vi "MakePlotDG535.vi"(5 "Polarity array":refnum<vi>[](array[refnum]), 6 "Amplitude array":refnum<vi>[](array[refnum]), 7 "Channel array":refnum<vi>[](array[refnum])) -> (0 "min value":dbl, 1 "Numeric 3":dbl, 2 "samples":i32, 3 "Numeric":T1 min=-999.0 max=999.0 format="%+.12f", 4 "Array":cluster{"Pulse Pattern":dbl[]}[](array[cluster]))   [LabVIEW 2013]
uses:
  GUI_DG645/DelayControl2.ctl
  <vilib>/Analysis/NI_AALBase.lvlib
panel:
  out "Pulse Pattern":dbl[](graph)
  out "Array 2":cluster{"Waveform Graph":dbl[]}[](array[cluster])
  out "Array 4":T1[](array[typedef]) min=-999.0 max=999.0 format="%+.12f"
  out "Array 3":dbl[](array[numeric])
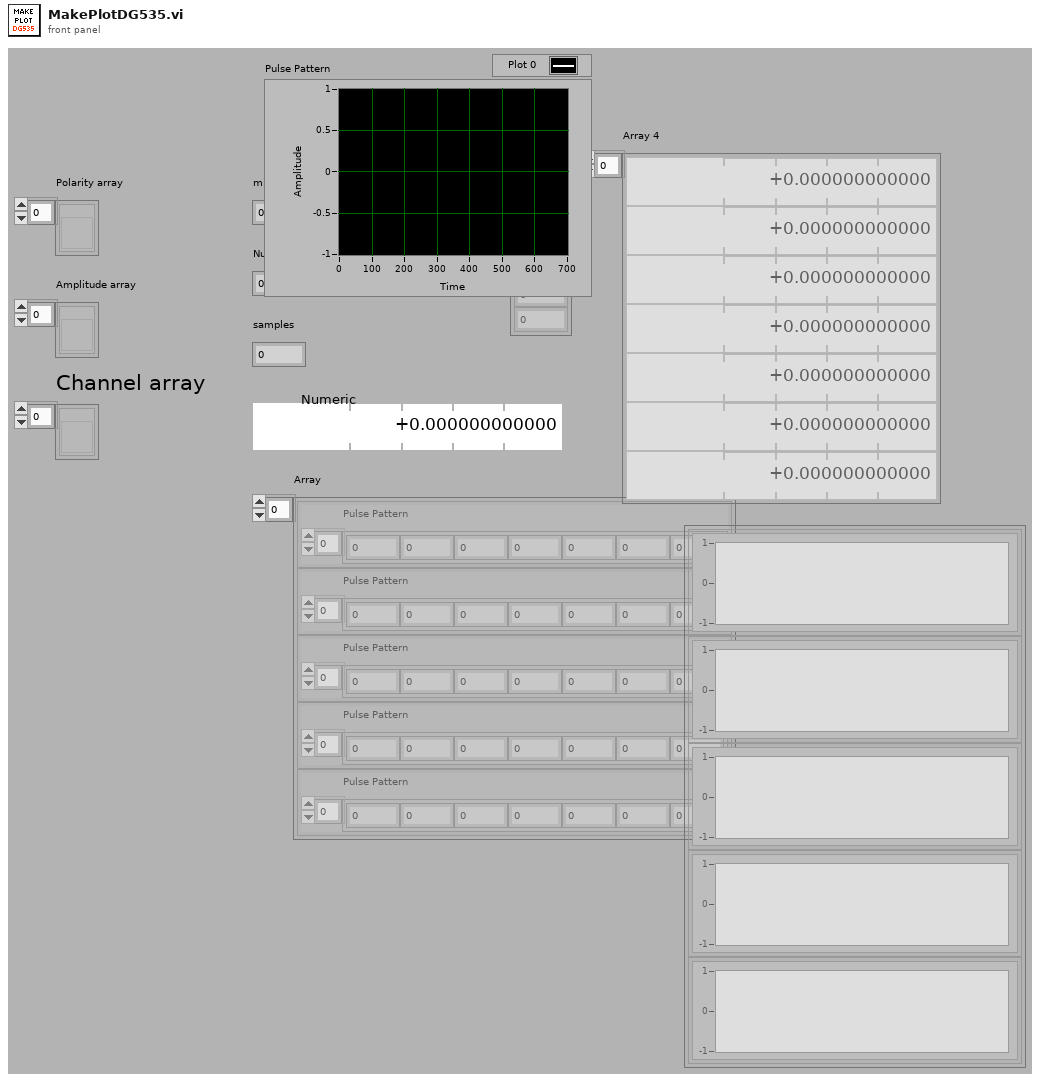
[diagram p1: front panel]
types:
  T1 = typedef "DelayControl2.ctl" = dbl
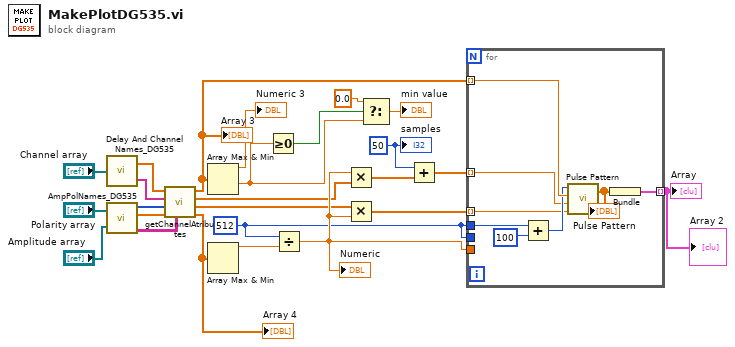
[diagram p0: block diagram]
diagram:
  w22 = 50 ("samples")
  w21 = 512 ("samples")
  n1 = call "Delay And Channel Names_DG535.vi"("Channel Array"="Channel array") -> ("Array"=w12:T1[], "Array 2"=w11:string[])
  n2 = call "AmpPolNames_DG535.vi"("Polarity array"="Polarity array", "Amplitude array"="Amplitude array") -> ("Array 2"=w9:enum16{"Negative", "Positive"}[], "Array 3"=w8:dbl[], "Array"=w10:string[][])  [unwired: 1 out]
  n3 = call "getChannelAtributes.vi"("Ch Name 2"=w10, "amplitude"=w8, "polarity"=w9, "Ch Name"=w11, "Delay"=w12) -> ("Array 4"=w14:T1[], "Array 2"=w16:T1[], "Array"=w18:T1[], "Array 3"=w15:dbl[])  [unwired: 1 in]
  "Array 3" <- w15
  "Array 4" <- w14
  n4 = Array Max & Min(array=w15) -> (max value=→"Numeric 3":dbl, min value=w3:dbl)  [unwired: 2 out]
  n5 = Array Max & Min(array=w14) -> (max value=w13:T1)  [unwired: 3 out]
  n6 = Greater Or Equal To 0?(x=w3) -> (x >= 0?=w5:bool)
  n7 = Divide(x=w21, y=w13) -> (x/y=w23:T1)
  "Numeric" <- w23
  n8 = Multiply(x=w23, y=w18) -> (x*y=w19:T1[])
  n9 = Multiply(x=w16, y=w23) -> (x*y=w17:T1[])
  n10 = Select(t=0.0, s=w5, f=w3) -> (s? t:f=→"min value":dbl)
  n11 = Add(x=w22, y=w19) -> (x+y=w20:T1[])
  n12 = for {
    tunnel: w21 -> [_]
    tunnel: w15 -> [w33] mode=indexing
    tunnel: w17 -> [w28] mode=indexing
    tunnel: [w31] -> w1 mode=indexing
    tunnel: w23 -> [_]
    tunnel: w20 -> [w27] mode=indexing
    tunnel: w21 -> [w26]
    n13 = Add(x=w26, y=100) -> (x+y=w30:i32)
    n14 = call <vilib>:"Pulse Pattern.vi"("width"=w28, "delay"=w27, "amplitude"=w33, "samples"=w30) -> ("Pulse Pattern"=w32:dbl[])  [unwired: 1 out]
    "Pulse Pattern" <- w32
    n15 = Bundle("Pulse Pattern"=w32) -> (w31:cluster{"Pulse Pattern":dbl[]})  [unwired: 1 in]
  }
  "Array" <- w1
  "Array 2" <- w1
  "samples" <- w22
